vi "Y_Jog_Plus.vi"() -> (3 "Final Y":sgl)   [LabVIEW 2013]
panel:
  in  "MG17Motor 3":refnum<k7>(container)
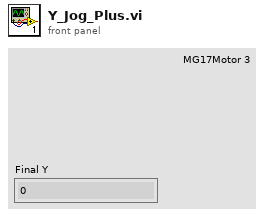
[diagram p1: front panel]
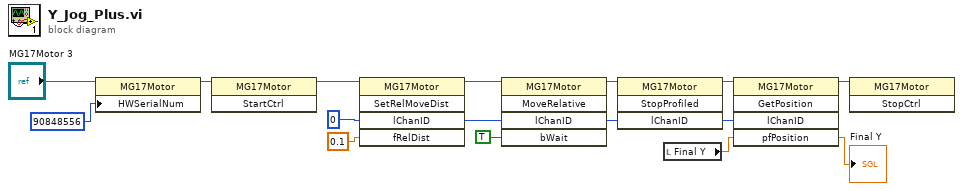
[diagram p0: block diagram]
diagram:
  n1 = property class="MG17Motor"(reference="MG17Motor 3", "HWSerialNum"=90848556 ("lChanID")) -> (reference out=w15:refnum<k7>)  [unwired: 1 in, 1 out]
  n2 = invoke class="MG17Motor" method="StartCtrl"(reference=w15) -> (reference out=w1:refnum<k7>)  [unwired: 2 in, 2 out]
  n3 = invoke class="MG17Motor" method="SetRelMoveDist"(reference=w1, "lChanID"=0, "fRelDist"=0.1) -> (reference out=w6:refnum<k7>, "lChanID"=w7:i32)  [unwired: 2 in, 3 out]
  n4 = invoke class="MG17Motor" method="MoveRelative"(reference=w6, "lChanID"=w7, "bWait"=TRUE) -> (reference out=w8:refnum<k7>, "lChanID"=w9:i32)  [unwired: 2 in, 3 out]
  n5 = invoke class="MG17Motor" method="StopProfiled"(reference=w8, "lChanID"=w9) -> (reference out=w12:refnum<k7>, "lChanID"=w10:i32)  [unwired: 2 in, 2 out]
  n6 = local read "Final Y"() -> (w13:sgl)
  n7 = invoke class="MG17Motor" method="GetPosition"(reference=w12, "lChanID"=w10, "pfPosition"=w13) -> (reference out=w11:refnum<k7>, "pfPosition"=→"Final Y":sgl)  [unwired: 2 in, 3 out]
  n8 = invoke class="MG17Motor" method="StopCtrl"(reference=w11) -> ()  [unwired: 2 in, 3 out]
